vi "Insert_Into_Array_1D.vi"(7 "E or S IIA":T1, 8 "SubArray IIA":i8[](array[numeric])=[-1, -2], 9 "Element IIA":i8, 10 "Index IIA":i32, 11 "Insert Into Array 1D":i8[](array[numeric])=[1, 2, 3, 4]) -> (3 "Array 1D IIA":i8[](array[numeric])=[1, 2, 3, 4])   [LabVIEW 2018]
uses:
  Controls/E_S.ctl
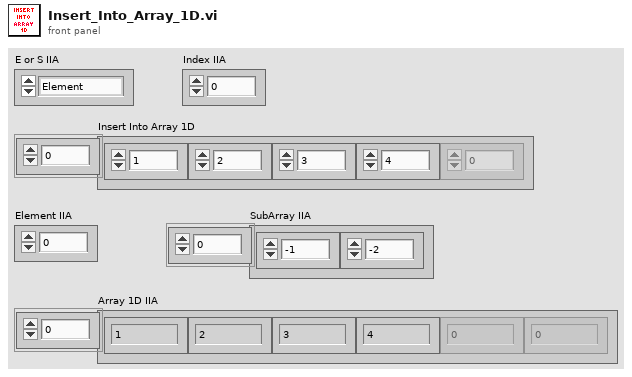
[diagram p1: front panel]
types:
  T1 = typedef "E_S.ctl" = enum16{"Element", "SubArray"}
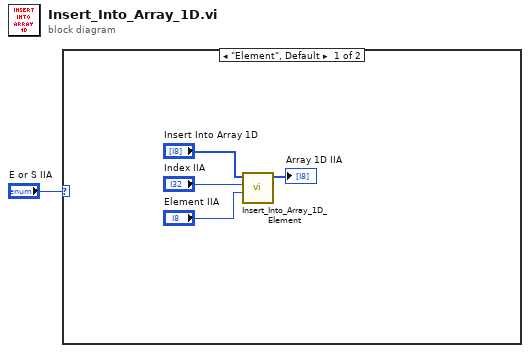
[diagram p0: block diagram]
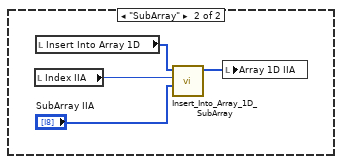
[diagram p2: hidden frame]
diagram:
  n1 = case shown="\"Element\", Default" "E or S IIA" {
    frame "Element", Default {
      n2 = call "Insert_Into_Array_1D_Element.vi"("Element IIA"="Element IIA", "Index IIA"="Index IIA", "Insert Into Array 1D"="Insert Into Array 1D") -> ("Array 1D IIA"=→"Array 1D IIA":i8[])  [unwired: 8 in]
    }
    frame "SubArray" {
      n3 = local read "Index IIA"() -> (w7:i32)
      n4 = local read "Insert Into Array 1D"() -> (w8:i8[])
      n5 = call "Insert_Into_Array_1D_SubArray.vi"("SubArray IIA"="SubArray IIA", "Index IIA"=w7, "Insert into Array 1D"=w8) -> ("Array 1D IIA"=w9:i8[])  [unwired: 8 in]
      n6 = local write "Array 1D IIA"(w9) -> ()
    }
  }
